vi "GET_character_by_id.vi"(8 "error in (no error)":errorcluster, 10 "character id":i32, 11 "REST Client in":refnum<class "REST Client.lvclass">) -> (0 "error out":errorcluster, 2 "local storyArc":T1, 3 "REST Client out":refnum<class "REST Client.lvclass">)   [LabVIEW 2024]
uses:
  <vilib>/addons/_JKI.lib/REST Client/classes/REST Client/REST Client.lvclass
  definitions/local_character.ctl
  <vilib>/addons/_JKI.lib/REST Client/classes/REST Client/HTTP Header.ctl
  <vilib>/NI/Advanced HTTP Client/Header--Combo Box.ctl
  definitions/comicvine_character.ctl
  definitions/comicvine_character.results.ctl
  definitions/comicvine_volume.issue.ctl
  definitions/comicvine_volume.publisher.ctl
  <vilib>/NI/Advanced HTTP Client/Session.lvclass
  <userlib>/_OpenG.lib/string/string.llb/openg_string.lvlib
  <vilib>/addons/_JKI.lib/Serialization/JSON/JKI JSON Serialization.lvlib
panel:
  out "Status String":string
  out "Status Code":u16
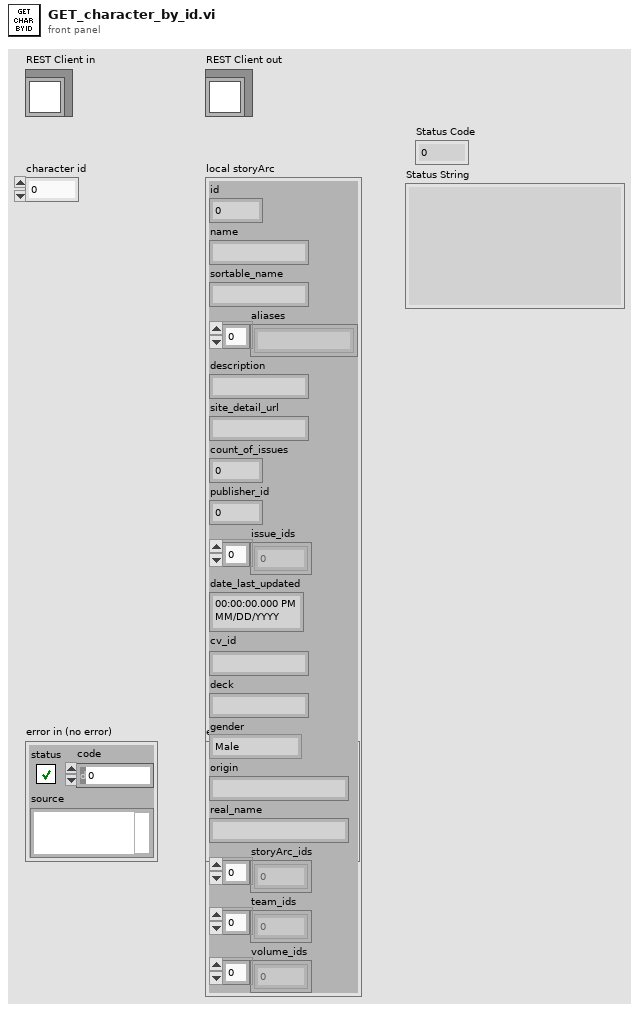
[diagram p1: front panel]
types:
  T1 = typedef "local_character.ctl" = cluster{"id":i32, "name":string, "sortable_name":string, "aliases":string[], "description":string, "site_detail_url":string, "count_of_issues":i32, "publisher_id":i32, "issue_ids":i32[], "date_last_updated":timestamp, "cv_id":string, "deck":string, "gender":enum16{"Male", "Female", "Other"}, "origin":string, "real_name":string, "storyArc_ids":i32[], "team_ids":i32[], "volume_ids":i32[]}
  T2 = typedef "comicvine_character.ctl" = cluster{"error":string, "limit":i32, "offset":i32, "number_of_page_results":i32, "number_of_total_results":i32, "status_code":i32, "results":T3}
  T3 = typedef "comicvine_character.results.ctl" = cluster{"aliases":string, "count_of_issue_appearances":i32, "date_last_updated":timestamp, "deck":string, "description":string, "gender":enum16{"Male", "Female", "Other"}, "id":i32, "issue_credits":T4[], "name":string, "origin":string, "publisher":T5, "real_name":string, "site_detail_url":string, "story_arc_credits":T4[], "teams":T4[], "volume_credits":T4[]}
  T4 = typedef "comicvine_volume.issue.ctl" = cluster{"id":i32}
  T5 = typedef "comicvine_volume.publisher.ctl" = cluster{"id":i32}
  T6 = typedef "REST Client.lvlib/REST Client.lvclass/HTTP Header.ctl" = cluster{"header":T7, "value":string}
  T7 = typedef "lib_NI_Advanced HTTP Client.lvlib/Session.lvclass/Header--Combo Box.ctl" = string
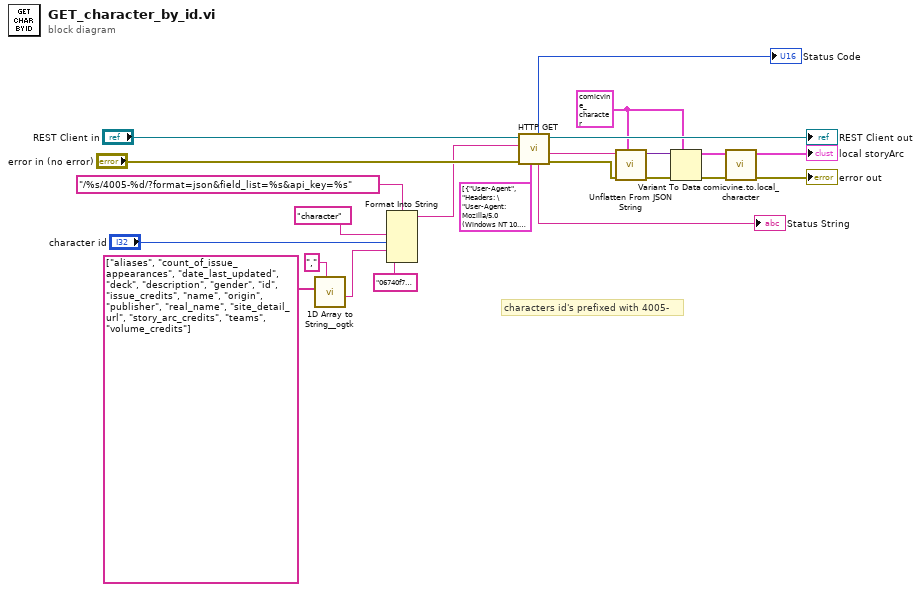
[diagram p0: block diagram]
diagram:
  w2 = T2 {"error"="", "limit"=0, "offset"=0, "number_of_page_results"=0, "number_of_total_results"=0, "status_code"=0, "results"={"aliases"="", "count_of_issue_appearances"=0, "date_last_updated"=timestamp(0 s since 1904-01-01), "deck"="", "description"="", "gender"=enum."Male", "id"=0, "issue_credits"=[], "name"="", "origin"="", "publisher"={"id"=0}, "real_name"="", "site_detail_url"="", "story_arc_credits"=[], "teams"=[], "volume_credits"=[]}} ("team")
  # "characters id's prefixed with 4005-"
  n1 = call <userlib>:"1D Array to String__ogtk.vi"("delimiter (Tab)"=",", "Array of Strings"=string[] ["aliases", "count_of_issue_appearances", "date_last_updated", "deck", "description", "gender", "id", "issue_credits", "name", "origin", "publisher", "real_name", "site_detail_url", "story_arc_credits", "teams", "volume_credits"]) -> ("delimited string"=w13:string)  [unwired: 9 in]
  n2 = Format Into String(format string="/%s/4005-%d/?format=json&field_list=%s&api_key=%s", "character" ("resource"), "character id", w13, "06740f73403e0b211d597c50ea94c7f16ea5e8ea") -> (resulting string=w18:string)  [unwired: 2 in, 1 out]
  n3 = call-dynamic "HTTP GET.vi"("request specific headers"=T6[] [{"header"="User-Agent", "value"="Headers: \"User-Agent: Mozilla/5.0 (Windows NT 10.0; Win64; x64) AppleWebKit/537.36 (KHTML, like Gecko) Chrome/91.0.4472.101 Safari/537.36\""}], "error in (no error)"="error in (no error)", "Path"=w18, "REST Client in"="REST Client in") -> ("error out"=w23:errorcluster, "Response body"=w12:string, "REST Client out"=→"REST Client out":refnum<class "REST Client.lvclass">, "Status String"=→"Status String":string, "Status Code"=→"Status Code":u16)  [unwired: 2 in, 1 out]
  n4 = call <vilib>:"Unflatten From JSON String.vi"("Type and Defaults"=w2, "error in"=w23, "JSON String"=w12) -> ("error out"=w10:errorcluster, "Variant"=w11:variant)  [unwired: 7 in]
  n5 = Variant To Data(error in=w10, type=w2, Variant=w11) -> (data=w7:T2, error out=w6:errorcluster)
  n6 = call "comicvine.to.local_character.vi"("error in (no error)"=w6, "cv character"=w7) -> ("error out"=→"error out":errorcluster, "local character"=→"local storyArc":T1)  [unwired: 8 in]
